vi "Unprocess Array Elements.vi"(6 "Variant Database":variant, 7 "Value":string, 8 "Error In":errorcluster, 9 "Name In":string, 10 "Array Variant":variant, 11 "Queue In":refnum<queue>) -> (0 "Error Out":errorcluster, 1 "Data Out":string, 3 "Queue Out":refnum<queue>)   [LabVIEW 2015]
doc: "This VI was created for use with the Read/Write Cluster VIs. It finds any array elements that have been written to file and places their value in the array.\n\nFreeware from Moore Good Ideas, www.mooregoodideas.com. Do not remove this line."
uses:
  <vilib>/Utility/VariantDataType/VariantType.lvlib
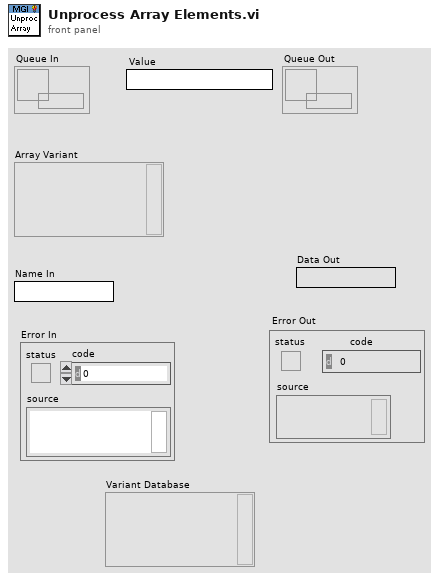
[diagram p1: front panel]
types:
  T1 = typedef "VariantType.lvlib/Type.ctl" = enum8{"Invalid Type", "Void", "I8", "I16", "I32", "I64", "U8", "U16", "U32", "U64", "Single Float", "Double Float", "Extended Float", "Single Complex", "Double Complex", "Extended Complex", "Enum U8", "Enum U16", "Enum U32", "Enum U64", "Single Float With Unit", "Double Float With Unit", "Extended Float With Unit", "Single Complex with Unit", "Double Complex with Unit", "Extended Complex with Unit", "Boolean", "String", "Path", "Picture", "Tag", "Array", "Cluster", "Variant", "LV Variant", "Waveform", "Timestamp", "Digital Waveform", "Digital Data", "ExpressData", "Refnum", "External Data", "VI", "Poly VI", "LabVIEW Class Instance", "Fixed Point"}
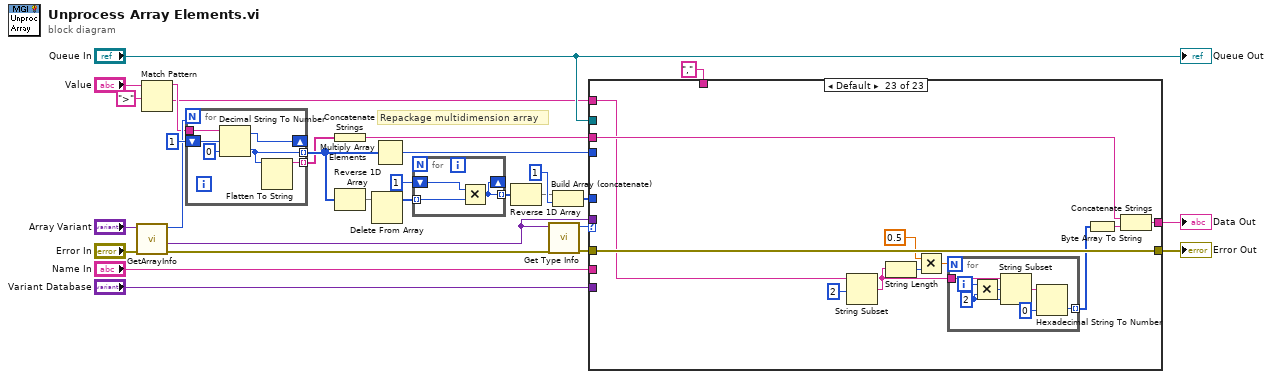
[diagram p0: block diagram]
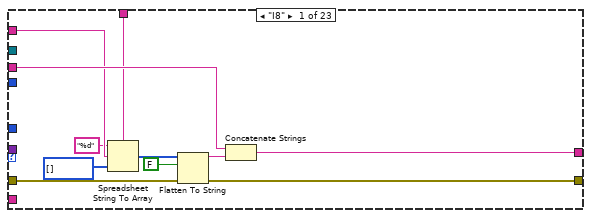
[diagram p2: hidden frame]
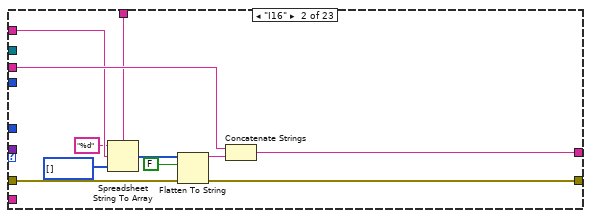
[diagram p3: hidden frame]
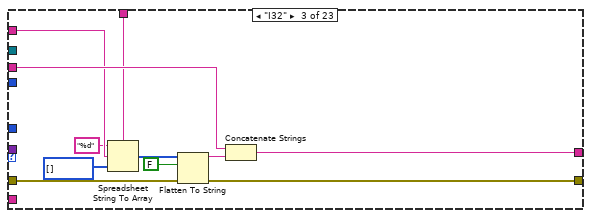
[diagram p4: hidden frame]
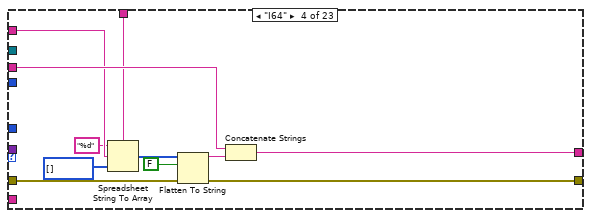
[diagram p5: hidden frame]
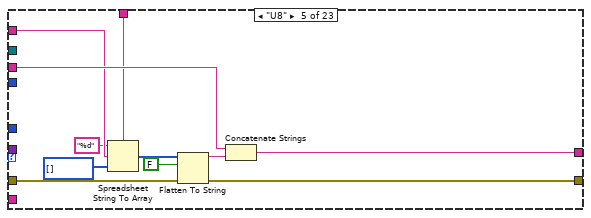
[diagram p6: hidden frame]
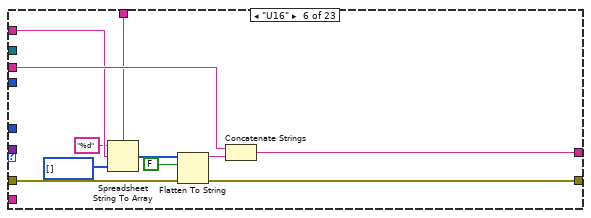
[diagram p7: hidden frame]
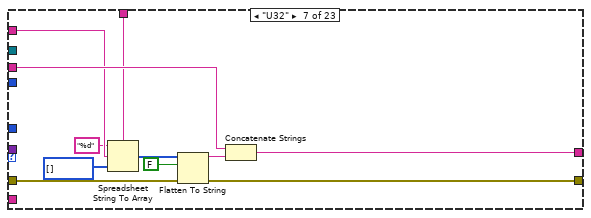
[diagram p8: hidden frame]
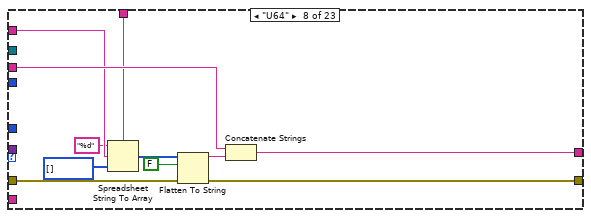
[diagram p9: hidden frame]
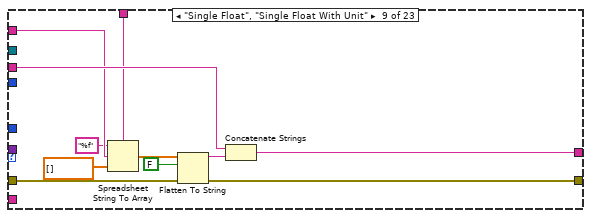
[diagram p10: hidden frame]
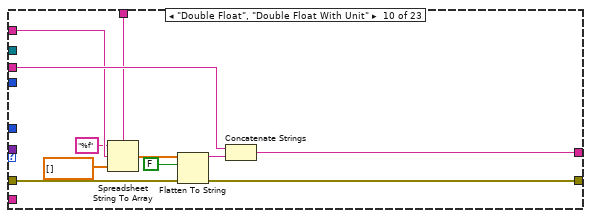
[diagram p11: hidden frame]
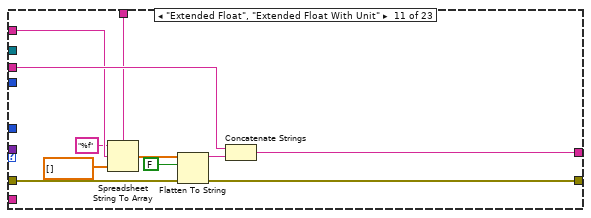
[diagram p12: hidden frame]
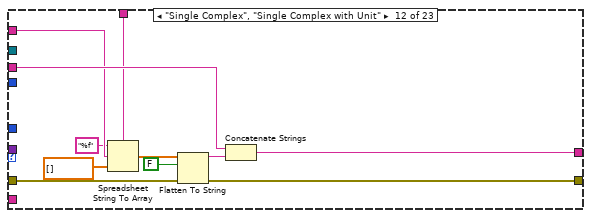
[diagram p13: hidden frame]
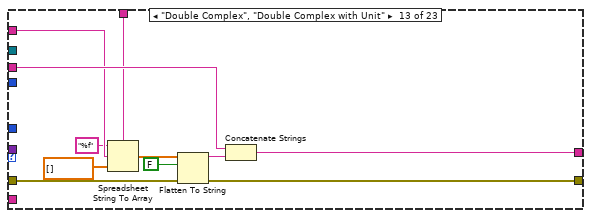
[diagram p14: hidden frame]
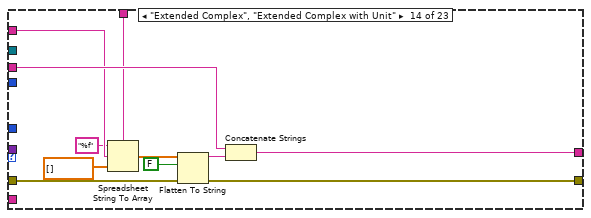
[diagram p15: hidden frame]
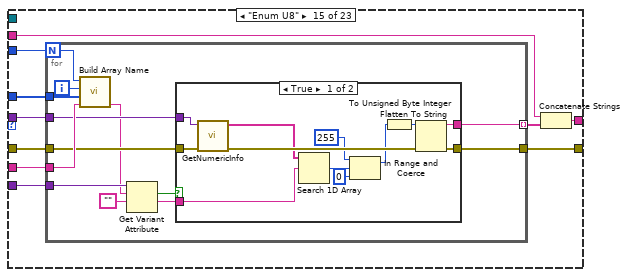
[diagram p16: hidden frame]
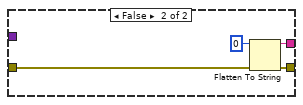
[diagram p17: hidden frame]
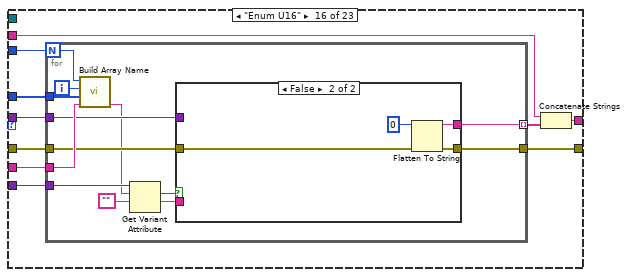
[diagram p18: hidden frame]
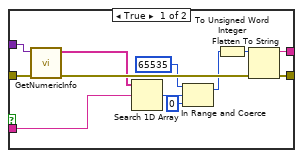
[diagram p19: hidden frame]
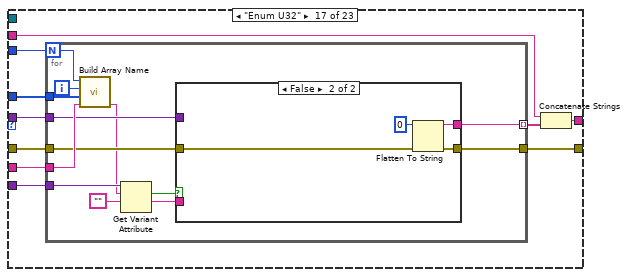
[diagram p20: hidden frame]
diagram:
  # "Repackage multidimension array"
  n1 = call <vilib>:"GetArrayInfo.vi"("error in (no error)"="Error In", "Variant"="Array Variant") -> ("error out"=w14:errorcluster, "ArrayElement"=w15:variant, "NDims"=w12:i32)  [unwired: 7 out]
  n2 = Match Pattern(string="Value", regular expression=">") -> (before substring=w5:string, after substring=w4:string)  [unwired: 3 out]
  n3 = for {
    N: w12 -> [_]
    shift-right: [w34] -> _
    shift-left: 1 ("offset past number") -> [w33]
    tunnel: w5 -> [w35]
    tunnel: [w31] -> w11 mode=indexing
    tunnel: [w30] -> w10 mode=indexing
    n4 = Decimal String To Number(string=w35, offset=w33, default (0L)=u32 0 ("default (0 I32)")) -> (offset past number=w34:i32, number=w31:u32)
    n5 = Flatten To String(anything=w31) -> (data string=w30:string)  [unwired: 1 in, 4 out]
  }
  n6 = Concatenate Strings(w10) -> (w9:string)
  n7 = Reverse 1D Array(array=w11) -> (reversed array=w19:u32[])
  n8 = Delete From Array(array=w19) -> (array with subset deleted=w20:u32[])  [unwired: 2 in, 1 out]
  n9 = Multiply Array Elements(1:w11) -> (0:w26:u32)
  n10 = for {
    tunnel: w20 -> [w38] mode=indexing
    shift-right: [w36] -> _
    shift-left: i8 1 -> [w37]
    tunnel: [w36] -> w22 mode=indexing
    n11 = Multiply(x=w37, y=w38) -> (x*y=w36:u32)
  }
  n12 = Reverse 1D Array(array=w22) -> (reversed array=w23:u32[])
  n13 = call "Get Type Info.vi"("Error In"=w14, "Variant"=w15) -> ("Error Out"=w27:errorcluster, "Type Enum"=w3:T1)  [unwired: 8 out]
  n14 = Build Array (concatenate)(w23, i8 1) -> (w18:u32[])
  n15 = case shown="Default" w3 {
    tunnel: [w49 w60 w71 w82 w93 w104 w115 w126 w137 w148 w159 w170 w181 w192 w202 w241 w280 w319 w357 w388 w417 w442 w474] -> w17
    tunnel: w27 -> [w48 w59 w70 w81 w92 w103 w114 w125 w136 w147 w158 w169 w180 w191 w201 w240 w279 w318 w356 w387 w416 w449 w474]
    tunnel: w9 -> [w46 w57 w68 w79 w90 w101 w112 w123 w134 w145 w156 w167 w178 w189 w195 w234 w273 w312 w350 w381 w410 w445 w472]
    tunnel: w26 -> [_ _ _ _ _ _ _ _ _ _ _ _ _ _ w200 w239 w278 w317 w355 w386 w415 w448 _]
    tunnel: "Name In" -> [_ _ _ _ _ _ _ _ _ _ _ _ _ _ w199 w238 w277 w316 w354 w385 w414 w447 _]
    tunnel: w18 -> [_ _ _ _ _ _ _ _ _ _ _ _ _ _ w198 w237 w276 w315 w353 w384 w413 w446 _]
    tunnel: "Queue In" -> [_ _ _ _ _ _ _ _ _ _ _ _ _ _ _ _ _ _ _ _ _ w441 _]
    tunnel: w15 -> [_ _ _ _ _ _ _ _ _ _ _ _ _ _ w193 w232 w271 w310 _ _ _ w444 _]
    tunnel: "Variant Database" -> [_ _ _ _ _ _ _ _ _ _ _ _ _ _ w197 w236 w275 w314 w352 w383 w412 _ _]
    tunnel: [w47 w58 w69 w80 w91 w102 w113 w124 w135 w146 w157 w168 w179 w190 w194 w233 w272 w311 w349 w380 w409 w445 w471] -> w8
    tunnel: w4 -> [w45 w56 w67 w78 w89 w100 w111 w122 w133 w144 w155 w166 w177 w188 _ _ _ _ _ _ _ _ w470]
    tunnel: "," ("delimiter (Tab)") -> [w39 w50 w61 w72 w83 w94 w105 w116 w127 w138 w149 w160 w171 w182 _ _ _ _ _ _ _ _ _]
    frame "I8" {
      n16 = Spreadsheet String To Array(delimiter (Tab)=w39, format string="%d", spreadsheet string=w45, array type (2D Dbl)=i8[] []) -> (array=w43:i8[])
      n17 = Flatten To String(anything=w43, prepend array or string size? (T)=FALSE, error in (no error)=w48) -> (data string=w40:string, error out=w49:errorcluster)  [unwired: 2 out]
      n18 = Concatenate Strings(w46, w40) -> (w47:string)
    }
    frame "I16" {
      n19 = Spreadsheet String To Array(delimiter (Tab)=w50, format string="%d", spreadsheet string=w56, array type (2D Dbl)=i16[] []) -> (array=w54:i16[])
      n20 = Flatten To String(anything=w54, prepend array or string size? (T)=FALSE, error in (no error)=w59) -> (data string=w51:string, error out=w60:errorcluster)  [unwired: 2 out]
      n21 = Concatenate Strings(w57, w51) -> (w58:string)
    }
    frame "I32" {
      n22 = Spreadsheet String To Array(delimiter (Tab)=w61, format string="%d", spreadsheet string=w67, array type (2D Dbl)=i32[] []) -> (array=w65:i32[])
      n23 = Flatten To String(anything=w65, prepend array or string size? (T)=FALSE, error in (no error)=w70) -> (data string=w62:string, error out=w71:errorcluster)  [unwired: 2 out]
      n24 = Concatenate Strings(w68, w62) -> (w69:string)
    }
    frame "I64" {
      n25 = Spreadsheet String To Array(delimiter (Tab)=w72, format string="%d", spreadsheet string=w78, array type (2D Dbl)=i64[] []) -> (array=w76:i64[])
      n26 = Flatten To String(anything=w76, prepend array or string size? (T)=FALSE, error in (no error)=w81) -> (data string=w73:string, error out=w82:errorcluster)  [unwired: 2 out]
      n27 = Concatenate Strings(w79, w73) -> (w80:string)
    }
    frame "U8" {
      n28 = Spreadsheet String To Array(delimiter (Tab)=w83, format string="%d", spreadsheet string=w89, array type (2D Dbl)=u8[] []) -> (array=w87:u8[])
      n29 = Flatten To String(anything=w87, prepend array or string size? (T)=FALSE, error in (no error)=w92) -> (data string=w84:string, error out=w93:errorcluster)  [unwired: 2 out]
      n30 = Concatenate Strings(w90, w84) -> (w91:string)
    }
    frame "U16" {
      n31 = Spreadsheet String To Array(delimiter (Tab)=w94, format string="%d", spreadsheet string=w100, array type (2D Dbl)=u16[] []) -> (array=w98:u16[])
      n32 = Flatten To String(anything=w98, prepend array or string size? (T)=FALSE, error in (no error)=w103) -> (data string=w95:string, error out=w104:errorcluster)  [unwired: 2 out]
      n33 = Concatenate Strings(w101, w95) -> (w102:string)
    }
    frame "U32" {
      n34 = Spreadsheet String To Array(delimiter (Tab)=w105, format string="%d", spreadsheet string=w111, array type (2D Dbl)=u32[] []) -> (array=w109:u32[])
      n35 = Flatten To String(anything=w109, prepend array or string size? (T)=FALSE, error in (no error)=w114) -> (data string=w106:string, error out=w115:errorcluster)  [unwired: 2 out]
      n36 = Concatenate Strings(w112, w106) -> (w113:string)
    }
    frame "U64" {
      n37 = Spreadsheet String To Array(delimiter (Tab)=w116, format string="%d", spreadsheet string=w122, array type (2D Dbl)=u64[] []) -> (array=w120:u64[])
      n38 = Flatten To String(anything=w120, prepend array or string size? (T)=FALSE, error in (no error)=w125) -> (data string=w117:string, error out=w126:errorcluster)  [unwired: 2 out]
      n39 = Concatenate Strings(w123, w117) -> (w124:string)
    }
    frame "Single Float", "Single Float With Unit" {
      n40 = Spreadsheet String To Array(delimiter (Tab)=w127, format string="%f", spreadsheet string=w133, array type (2D Dbl)=sgl[] []) -> (array=w131:sgl[])
      n41 = Flatten To String(anything=w131, prepend array or string size? (T)=FALSE, error in (no error)=w136) -> (data string=w128:string, error out=w137:errorcluster)  [unwired: 2 out]
      n42 = Concatenate Strings(w134, w128) -> (w135:string)
    }
    frame "Double Float", "Double Float With Unit" {
      n43 = Spreadsheet String To Array(delimiter (Tab)=w138, format string="%f", spreadsheet string=w144, array type (2D Dbl)=dbl[] []) -> (array=w142:dbl[])
      n44 = Flatten To String(anything=w142, prepend array or string size? (T)=FALSE, error in (no error)=w147) -> (data string=w139:string, error out=w148:errorcluster)  [unwired: 2 out]
      n45 = Concatenate Strings(w145, w139) -> (w146:string)
    }
    frame "Extended Float", "Extended Float With Unit" {
      n46 = Spreadsheet String To Array(delimiter (Tab)=w149, format string="%f", spreadsheet string=w155, array type (2D Dbl)=ext[] []) -> (array=w153:ext[])
      n47 = Flatten To String(anything=w153, prepend array or string size? (T)=FALSE, error in (no error)=w158) -> (data string=w150:string, error out=w159:errorcluster)  [unwired: 2 out]
      n48 = Concatenate Strings(w156, w150) -> (w157:string)
    }
    frame "Single Complex", "Single Complex with Unit" {
      n49 = Spreadsheet String To Array(delimiter (Tab)=w160, format string="%f", spreadsheet string=w166, array type (2D Dbl)=csg[] []) -> (array=w164:csg[])
      n50 = Flatten To String(anything=w164, prepend array or string size? (T)=FALSE, error in (no error)=w169) -> (data string=w161:string, error out=w170:errorcluster)  [unwired: 2 out]
      n51 = Concatenate Strings(w167, w161) -> (w168:string)
    }
    frame "Double Complex", "Double Complex with Unit" {
      n52 = Spreadsheet String To Array(delimiter (Tab)=w171, format string="%f", spreadsheet string=w177, array type (2D Dbl)=cdb[] []) -> (array=w175:cdb[])
      n53 = Flatten To String(anything=w175, prepend array or string size? (T)=FALSE, error in (no error)=w180) -> (data string=w172:string, error out=w181:errorcluster)  [unwired: 2 out]
      n54 = Concatenate Strings(w178, w172) -> (w179:string)
    }
    frame "Extended Complex", "Extended Complex with Unit" {
      n55 = Spreadsheet String To Array(delimiter (Tab)=w182, format string="%f", spreadsheet string=w188, array type (2D Dbl)=cxt[] []) -> (array=w186:cxt[])
      n56 = Flatten To String(anything=w186, prepend array or string size? (T)=FALSE, error in (no error)=w191) -> (data string=w183:string, error out=w192:errorcluster)  [unwired: 2 out]
      n57 = Concatenate Strings(w189, w183) -> (w190:string)
    }
    frame "Enum U8" {
      n58 = for {
        N: w200 -> [w215]
        tunnel: [w209] -> w202
        tunnel: w201 -> [w211]
        tunnel: w199 -> [w212]
        tunnel: w198 -> [w213]
        tunnel: w197 -> [w210]
        tunnel: [w208] -> w196 mode=indexing
        tunnel: w193 -> [w207]
        i -> [w214]
        n59 = call "Build Array Name.vi"("Name In"=w212, "Array"=w213, "Iteration"=w214, "Iterations"=w215) -> ("Name Out"=w206:string)  [unwired: 1 in, 6 out]
        n60 = Get Variant Attribute(Variant=w210, name=w206, default value (empty Variant)="") -> (found=w204:bool, value=w203:string)  [unwired: 1 in, 2 out]
        n61 = case shown="True" w204 {
          tunnel: [w226 w228] -> w209
          tunnel: w211 -> [w225 w229]
          tunnel: [w227 w231] -> w208
          tunnel: w207 -> [w224 _]
          tunnel: w203 -> [w216 _]
          frame True {
            n62 = call <vilib>:"GetNumericInfo.vi"("error in (no error)"=w225, "Variant"=w224) -> ("error out"=w223:errorcluster, "EnumNames"=w218:string[])  [unwired: 8 out]
            n63 = Search 1D Array(1D array=w218, element=w216) -> (index of element=w219:i32)  [unwired: 1 out]
            n64 = In Range and Coerce(upper limit=255, x=w219, lower limit=0) -> (coerced(x)=w217:i32)  [unwired: 1 out]
            n65 = To Unsigned Byte Integer(number=w217) -> (unsigned 8bit integer=w222:u8)
            n66 = Flatten To String(anything=w222, error in (no error)=w223) -> (data string=w227:string, error out=w226:errorcluster)  [unwired: 3 out]
          }
          frame False {
            n67 = Flatten To String(anything=u8 0, error in (no error)=w229) -> (data string=w231:string, error out=w228:errorcluster)  [unwired: 3 out]
          }
        }
      }
      n68 = Concatenate Strings(w195, w196) -> (w194:string)
    }
    frame "Enum U16" {
      n69 = for {
        N: w239 -> [w254]
        tunnel: [w249] -> w241
        tunnel: w240 -> [w250]
        tunnel: w238 -> [w251]
        tunnel: w237 -> [w252]
        tunnel: w236 -> [w244]
        tunnel: [w248] -> w235 mode=indexing
        tunnel: w232 -> [w247]
        i -> [w253]
        n70 = call "Build Array Name.vi"("Name In"=w251, "Array"=w252, "Iteration"=w253, "Iterations"=w254) -> ("Name Out"=w243:string)  [unwired: 1 in, 6 out]
        n71 = Get Variant Attribute(Variant=w244, name=w243, default value (empty Variant)="") -> (found=w245:bool, value=w242:string)  [unwired: 1 in, 2 out]
        n72 = case shown="False" w245 {
          tunnel: [w265 w267] -> w249
          tunnel: w250 -> [w264 w268]
          tunnel: [w266 w270] -> w248
          tunnel: w247 -> [w263 _]
          tunnel: w242 -> [w255 _]
          frame True {
            n73 = call <vilib>:"GetNumericInfo.vi"("error in (no error)"=w264, "Variant"=w263) -> ("error out"=w262:errorcluster, "EnumNames"=w257:string[])  [unwired: 8 out]
            n74 = Search 1D Array(1D array=w257, element=w255) -> (index of element=w258:i32)  [unwired: 1 out]
            n75 = In Range and Coerce(upper limit=65535, x=w258, lower limit=0) -> (coerced(x)=w256:i32)  [unwired: 1 out]
            n76 = To Unsigned Word Integer(number=w256) -> (unsigned 16bit integer=w261:u16)
            n77 = Flatten To String(anything=w261, error in (no error)=w262) -> (data string=w266:string, error out=w265:errorcluster)  [unwired: 3 out]
          }
          frame False {
            n78 = Flatten To String(anything=u16 0, error in (no error)=w268) -> (data string=w270:string, error out=w267:errorcluster)  [unwired: 3 out]
          }
        }
      }
      n79 = Concatenate Strings(w234, w235) -> (w233:string)
    }
    frame "Enum U32" {
      n80 = for {
        N: w278 -> [w293]
        tunnel: [w288] -> w280
        tunnel: w279 -> [w289]
        tunnel: w277 -> [w290]
        tunnel: w276 -> [w291]
        tunnel: w275 -> [w284]
        tunnel: [w287] -> w274 mode=indexing
        tunnel: w271 -> [w286]
        i -> [w292]
        n81 = call "Build Array Name.vi"("Name In"=w290, "Array"=w291, "Iteration"=w292, "Iterations"=w293) -> ("Name Out"=w282:string)  [unwired: 1 in, 6 out]
        n82 = Get Variant Attribute(Variant=w284, name=w282, default value (empty Variant)="") -> (found=w285:bool, value=w281:string)  [unwired: 1 in, 2 out]
        n83 = case shown="False" w285 {
          tunnel: [w304 w306] -> w288
          tunnel: w289 -> [w303 w307]
          tunnel: [w305 w309] -> w287
          tunnel: w286 -> [w302 _]
          tunnel: w281 -> [w294 _]
          frame True {
            n84 = call <vilib>:"GetNumericInfo.vi"("error in (no error)"=w303, "Variant"=w302) -> ("error out"=w301:errorcluster, "EnumNames"=w297:string[])  [unwired: 8 out]
            n85 = Search 1D Array(1D array=w297, element=w294) -> (index of element=w298:i32)  [unwired: 1 out]
            n86 = In Range and Coerce(upper limit=u32 4294967295, x=w298, lower limit=0) -> (coerced(x)=w296:u32)  [unwired: 1 out]
            n87 = To Unsigned Long Integer(number=w296) -> (unsigned 32bit integer=w300:u32)
            n88 = Flatten To String(anything=w300, error in (no error)=w301) -> (data string=w305:string, error out=w304:errorcluster)  [unwired: 3 out]
          }
          frame False {
            n89 = Flatten To String(anything=u32 0, error in (no error)=w307) -> (data string=w309:string, error out=w306:errorcluster)  [unwired: 3 out]
          }
        }
      }
      n90 = Concatenate Strings(w273, w274) -> (w272:string)
    }
    frame "Enum U64" {
      n91 = for {
        N: w317 -> [w332]
        tunnel: [w327] -> w319
        tunnel: w318 -> [w328]
        tunnel: w316 -> [w329]
        tunnel: w315 -> [w330]
        tunnel: w314 -> [w322]
        tunnel: [w326] -> w313 mode=indexing
        tunnel: w310 -> [w325]
        i -> [w331]
        n92 = call "Build Array Name.vi"("Name In"=w329, "Array"=w330, "Iteration"=w331, "Iterations"=w332) -> ("Name Out"=w321:string)  [unwired: 1 in, 6 out]
        n93 = Get Variant Attribute(Variant=w322, name=w321, default value (empty Variant)="") -> (found=w323:bool, value=w320:string)  [unwired: 1 in, 2 out]
        n94 = case shown="False" w323 {
          tunnel: [w343 w345] -> w327
          tunnel: w328 -> [w342 w346]
          tunnel: [w344 w348] -> w326
          tunnel: w325 -> [w341 _]
          tunnel: w320 -> [w333 _]
          frame True {
            n95 = call <vilib>:"GetNumericInfo.vi"("error in (no error)"=w342, "Variant"=w341) -> ("error out"=w340:errorcluster, "EnumNames"=w336:string[])  [unwired: 8 out]
            n96 = Search 1D Array(1D array=w336, element=w333) -> (index of element=w337:i32)  [unwired: 1 out]
            n97 = In Range and Coerce(upper limit=u64 18446744073709551615, x=w337, lower limit=0) -> (coerced(x)=w335:u64)  [unwired: 1 out]
            n98 = To Unsigned Quad Integer(1:w335) -> (0:w339:u64)
            n99 = Flatten To String(anything=w339, error in (no error)=w340) -> (data string=w344:string, error out=w343:errorcluster)  [unwired: 3 out]
          }
          frame False {
            n100 = Flatten To String(anything=u64 0, error in (no error)=w346) -> (data string=w348:string, error out=w345:errorcluster)  [unwired: 3 out]
          }
        }
      }
      n101 = Concatenate Strings(w312, w313) -> (w311:string)
    }
    frame "Boolean" {
      n102 = for {
        N: w355 -> [w369]
        tunnel: [w364] -> w357
        tunnel: w356 -> [w365]
        tunnel: w354 -> [w366]
        tunnel: w353 -> [w367]
        tunnel: w352 -> [w360]
        tunnel: [w363] -> w351 mode=indexing
        i -> [w368]
        n103 = call "Build Array Name.vi"("Name In"=w366, "Array"=w367, "Iteration"=w368, "Iterations"=w369) -> ("Name Out"=w359:string)  [unwired: 1 in, 6 out]
        n104 = Get Variant Attribute(Variant=w360, name=w359, default value (empty Variant)="") -> (found=w361:bool, value=w358:string)  [unwired: 1 in, 2 out]
        n105 = case shown="True" w361 {
          tunnel: [w374 w377] -> w364
          tunnel: w365 -> [w373 w378]
          tunnel: [w375 w379] -> w363
          tunnel: w358 -> [w370 _]
          frame True {
            n106 = Equal?(x=w370, y="TRUE") -> (x = y?=w371:bool)
            n107 = Flatten To String(anything=w371, error in (no error)=w373) -> (data string=w375:string, error out=w374:errorcluster)  [unwired: 3 out]
          }
          frame False {
            n108 = Flatten To String(anything=FALSE, error in (no error)=w378) -> (data string=w379:string, error out=w377:errorcluster)  [unwired: 3 out]
          }
        }
      }
      n109 = Concatenate Strings(w350, w351) -> (w349:string)
    }
    frame "String" {
      n110 = for {
        N: w386 -> [w400]
        tunnel: [w395] -> w388
        tunnel: w387 -> [w396]
        tunnel: w385 -> [w397]
        tunnel: w384 -> [w398]
        tunnel: w383 -> [w391]
        tunnel: [w394] -> w382 mode=indexing
        i -> [w399]
        n111 = call "Build Array Name.vi"("Name In"=w397, "Array"=w398, "Iteration"=w399, "Iterations"=w400) -> ("Name Out"=w390:string)  [unwired: 1 in, 6 out]
        n112 = Get Variant Attribute(Variant=w391, name=w390, default value (empty Variant)="") -> (found=w392:bool, value=w389:string)  [unwired: 1 in, 2 out]
        n113 = case shown="False" w392 {
          tunnel: [w403 w406] -> w395
          tunnel: w396 -> [w402 w407]
          tunnel: [w404 w408] -> w394
          tunnel: w389 -> [w401 _]
          frame True {
            n114 = Flatten To String(anything=w401, error in (no error)=w402) -> (data string=w404:string, error out=w403:errorcluster)  [unwired: 3 out]
          }
          frame False {
            n115 = Flatten To String(anything="", error in (no error)=w407) -> (data string=w408:string, error out=w406:errorcluster)  [unwired: 3 out]
          }
        }
      }
      n116 = Concatenate Strings(w381, w382) -> (w380:string)
    }
    frame "Path" {
      n117 = for {
        N: w415 -> [w429]
        tunnel: [w424] -> w417
        tunnel: w416 -> [w425]
        tunnel: w414 -> [w426]
        tunnel: w413 -> [w427]
        tunnel: w412 -> [w421]
        tunnel: [w423] -> w411 mode=indexing
        i -> [w428]
        n118 = call "Build Array Name.vi"("Name In"=w426, "Array"=w427, "Iteration"=w428, "Iterations"=w429) -> ("Name Out"=w420:string)  [unwired: 1 in, 6 out]
        n119 = Get Variant Attribute(Variant=w421, name=w420, default value (empty Variant)="") -> (found=w419:bool, value=w418:string)  [unwired: 1 in, 2 out]
        n120 = case shown="False" w419 {
          tunnel: [w433 w436] -> w424
          tunnel: w425 -> [w432 w437]
          tunnel: [w434 w438] -> w423
          tunnel: w418 -> [w430 _]
          frame True {
            n121 = String To Path(string=w430) -> (path=w431:path)
            n122 = Flatten To String(anything=w431, error in (no error)=w432) -> (data string=w434:string, error out=w433:errorcluster)  [unwired: 3 out]
          }
          frame False {
            n123 = Flatten To String(anything=path "", error in (no error)=w437) -> (data string=w438:string, error out=w436:errorcluster)  [unwired: 3 out]
          }
        }
      }
      n124 = Concatenate Strings(w410, w411) -> (w409:string)
    }
    frame "Cluster" {
      # "Enqueue cluster element"
      n125 = for {
        N: w448 -> [w463]
        tunnel: w449 -> [w455]
        tunnel: w447 -> [w460]
        tunnel: w446 -> [w461]
        tunnel: w444 -> [w456]
        tunnel: [w455] -> w443
        tunnel: [w454] -> w440 mode=indexing
        i -> [w462]
        n126 = call "Build Array Name.vi"("Name In"=w460, "Array"=w461, "Iteration"=w462, "Iterations"=w463) -> ("Name Out"=w457:string)  [unwired: 1 in, 6 out]
        n127 = Concatenate Strings(w457, "." ("string")) -> (w459:string)
        n128 = Bundle("ArrayElement"=w456, w459) -> (w454:cluster{"ArrayElement":variant, string})  [unwired: 1 out]
      }
      n129 = Reverse 1D Array(array=w440) -> (reversed array=w439:cluster{"ArrayElement":variant, string}[])
      n130 = for {
        tunnel: w443 -> [w453]
        tunnel: [w452] -> w442
        tunnel: w441 -> [w451]
        tunnel: w439 -> [w450] mode=indexing
        n131 = Enqueue Element At Opposite End(queue=w451, element=w450, error in (no error)=w453) -> (error out=w452:errorcluster)  [unwired: 3 out]
      }
    }
    frame Default {
      n132 = String Subset(string=w470, offset (0)=2) -> (substring=w467:string)  [unwired: 1 out]
      n133 = String Length(string=w467) -> (length=w468:i32)
      n134 = Multiply(x=0.5, y=w468) -> (x*y=w469:dbl)
      n135 = for {
        N: w469 -> [_]
        tunnel: w467 -> [w478]
        tunnel: [w480] -> w465 mode=indexing
        i -> [w477]
        w476 = 2 ("length (rest)")
        n136 = Multiply(x=w477, y=w476) -> (x*y=w475:i32)
        n137 = String Subset(string=w478, offset (0)=w475, length (rest)=w476) -> (substring=w479:string)
        n138 = Hexadecimal String To Number(string=w479, default (0uL)=u8 0 ("default (0 U32)")) -> (number=w480:u8)  [unwired: 2 out]
      }
      n139 = Byte Array To String(unsigned byte array=w465) -> (string=w473:string)
      n140 = Concatenate Strings(w472, w473) -> (w471:string)
    }
  }
  "Error Out" <- w17
  "Data Out" <- w8
  "Queue Out" <- "Queue In"
